vi "Tank (reentrant).vi"() -> ()   [LabVIEW 2011]
panel:
  in  "stop":bool
  out "Tank":dbl(slide) scale=0.0..10.0
  # "This is a reentrant VI"
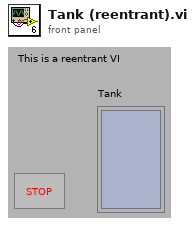
[diagram p1: front panel]
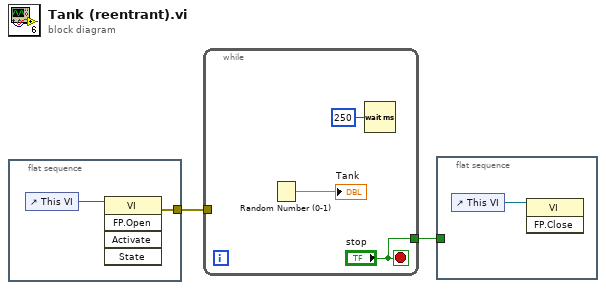
[diagram p0: block diagram]
diagram:
  n1 = flat-sequence {
    tunnel: [w3] -> w1
    frame #0 {
      n2 = control-ref of="This VI"() -> (w4:refnum<vi>)
      n3 = invoke class="VI" method="FP.Open"(reference=w4) -> (error out=w3:errorcluster)  [unwired: 4 in, 4 out]
    }
  }
  n4 = while {
    tunnel: ["stop"] -> w2
    tunnel: w1 -> [_]
    stop <- "stop" stop-if-true
    n5 = Random Number (0-1)() -> (number: 0 to 1=→"Tank":dbl)
    n6 = Wait (ms)(milliseconds to wait=u32 250 ("millisecond multiple")) -> ()  [unwired: 1 out]
  }
  n7 = flat-sequence {
    tunnel: w2 -> [_]
    frame #0 {
      n8 = control-ref of="This VI"() -> (w8:refnum<vi>)
      n9 = invoke class="VI" method="FP.Close"(reference=w8) -> ()  [unwired: 2 in, 3 out]
    }
  }
